vi "Read Data Model.vi"(8 "error in (no error)":errorcluster, 11 "Master CR in":refnum<class "WebSocket Client CR.lvclass">) -> (0 "error out":errorcluster, 2 "Data Model":refnum<class "Device Data Model.lvclass">, 3 "Master CR out":refnum<class "WebSocket Client CR.lvclass">)   [LabVIEW 2021, in "WebSockets.lvlib" / "WebSocket Client CR.lvclass"]
uses:
  WebSocket Client CR.lvclass
  Modbus_v121c/Data Model/Device Data Model.lvclass
  WebSocket Client CR.lvclass/WebSocket Client CR.ctl
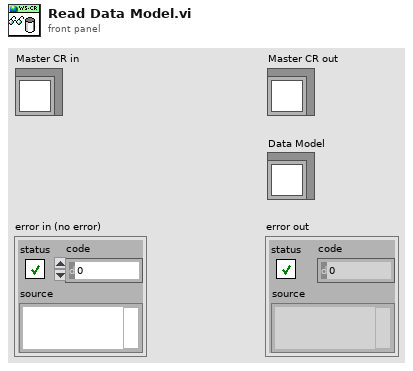
[diagram p1: front panel]
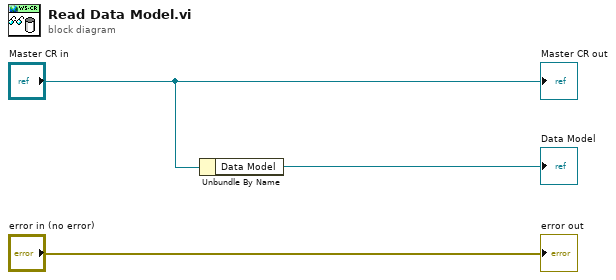
[diagram p0: block diagram]
diagram:
  n1 = Unbundle By Name("Master CR in") -> ("Data Model"=→"Data Model":refnum<class "Device Data Model.lvclass">)
  "error out" <- "error in (no error)"
  "Master CR out" <- "Master CR in"
